vi "Automotive ECU - Park Brake.vi"() -> ()   [LabVIEW 2013]
doc: "Sample numeric display item."
uses:
  <vilib>/NI Veristand/Display Template Support/Display Template Support.llb/cluster_Screen Item Settings.ctl
  <vilib>/NI Veristand/Display Template Support/Display Template Support.llb/cluster_Graph Scale Settings.ctl
  <vilib>/NI Veristand/Display Template Support/Display Template Support.llb/cluster_Graph Plot Settings.ctl
  NationalInstruments.VeriStand.SystemStorage
  <vilib>/NI Veristand/Display Template Support/Display Template Support.llb/enum_Display Template Handler Minimal To Widget Msg.ctl
  <vilib>/NI Veristand/Display Template Support/Display Template Support.llb/enum_Display Template Handler Minimal To Workspace.ctl
  Support/Parking Brake Parameters.ctl
  <vilib>/NI Veristand/Execution/Workspace/NI_VS Workspace ExecutionAPI.lvlib
panel:
  in  "Parked":bool
  out "Label":string="Numeric"
  out "Status Indicator":string
  in  "NIVS.System Definition Root":refnum<k24>
  in  "NIVS.Gateway IP Address":string
  in  "Item.Data":T1
  # "Status:"
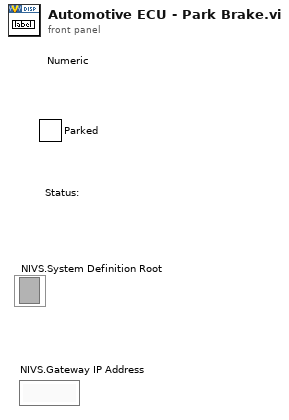
[diagram p1: front panel]
types:
  T1 = typedef "cluster_Screen Item Settings.ctl" = cluster{"Template VI":string, "Position X":i32, "Position Y":i32, "Custom":string, "Show Title Bar":bool, "ID":i32, "Always On Top":bool, "Allow Resize":bool, "Allow Minimize":bool, "Allow Close":bool, "Size to Screen":bool, "Screen.ID":i32, "State":enum16{"Normal", "New"}, "Title":string, "Window Bounds":cluster{"[0]":i16, "[1]":i16, "[2]":i16, "[3]":i16}, "Channel Ref":u64, "Unit":string, "Default Units?":bool, "Flash Limit?":bool, "Color 1":u32, "Color 2":u32, "Color 3":u32, "Color 4":u32, "Bck Color":u32, "Fore Color":u32, "Limit 1":dbl, "Limit 2":dbl, "Limit 3":dbl, "Limit 4":dbl, "Limit Mode 1":i32, "Limit Mode 2":i32, "Limit Mode 3":i32, "Limit Mode 4":i32, "Scale Precision":i32, "Scale Min":dbl, "Scale Max":dbl, "Format":i32, "Precision":i32, "Background Type":i32, "IDs":i32[], "Units":string[], "Labels":string[], "Scale Factor":dbl, "Scale Offset":dbl, "YScale Index":u32[], "XScale":T2, "YScales":T2[], "Plots":T3[], "Update Period":dbl, "History Length":dbl, "My.Ref":refnum<vi>, "Is Control?":bool, "Channel Paths":string[], "Custom Data":variant}
  T2 = typedef "cluster_Graph Scale Settings.ctl" = cluster{"Format":u8, "Precision":u8, "Fit":u8, "Label":string, "Use Default Label":bool, "Label Visible":bool, "Min":dbl, "Max":dbl}
  T3 = typedef "cluster_Graph Plot Settings.ctl" = cluster{"Bar Style":u8, "Fill To":i16, "Fill/PtColor":u32, "Line Style":u8, "Line Width":u8, "Color":u32, "Interp":u8, "Point Style":u8}
  T4 = typedef "enum_Display Template Handler Minimal To Workspace.ctl" = cluster{"Operation":enum16{"SetCustomData", "DeleteItem"}, "Data":variant}
  T5 = typedef "enum_Display Template Handler Minimal To Widget Msg.ctl" = enum16{"Stop", "LaunchConfigDialog"}
  T6 = typedef "Parking Brake Parameters.ctl" = cluster{"Ground on Engage":cluster{"Path Array":string[], "Node Path":string}, "Ground on Disengage":cluster{"Path Array":string[], "Node Path":string}, "Lower Pane Color":u32, "Upper Pane Color":u32, "Initialized?":bool, "Label":string}
  T7 = typedef "NI_VS Workspace ExecutionAPI.lvlib/WorkspaceAPI.ctl" = refnum<k24>
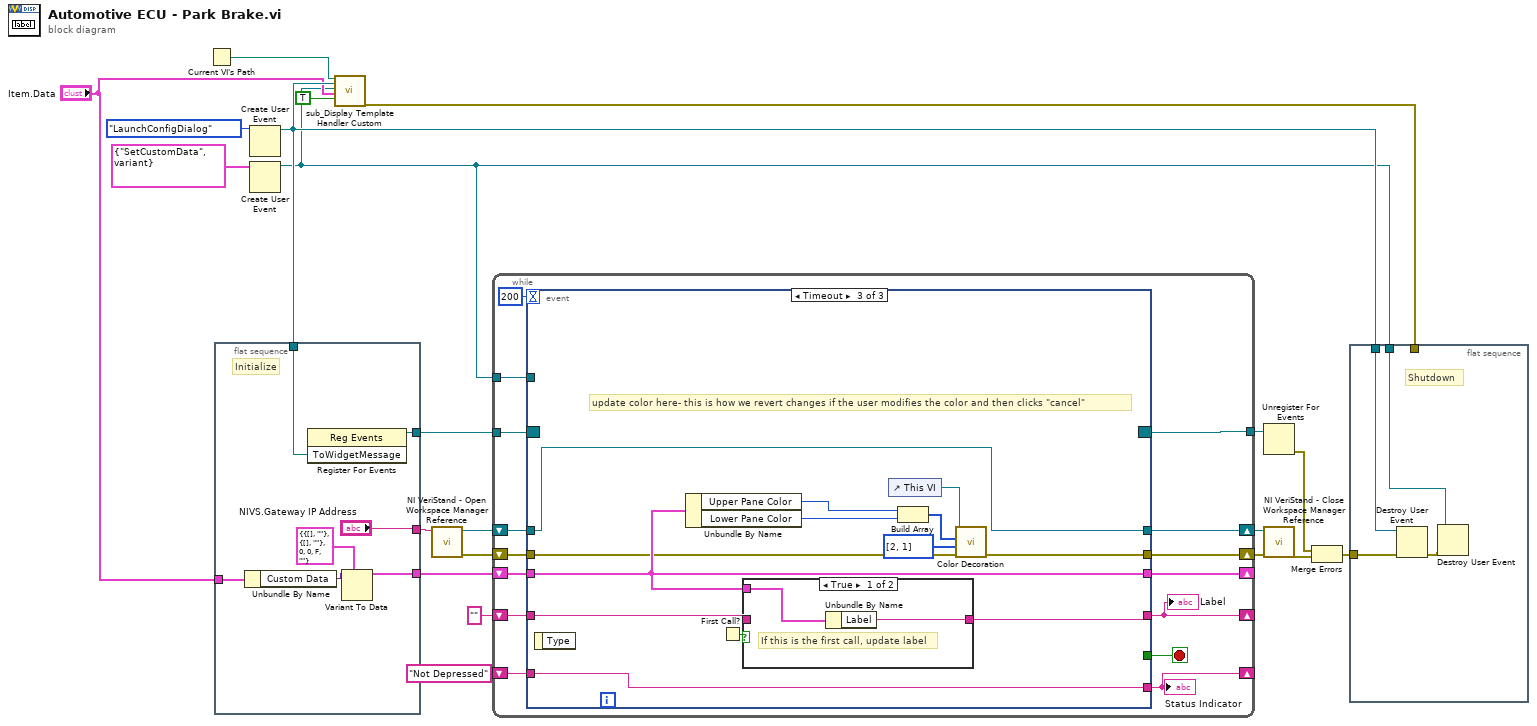
[diagram p0: block diagram]
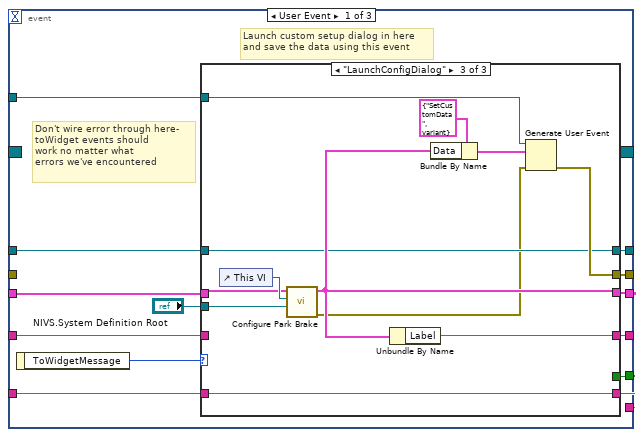
[diagram p2: hidden frame]
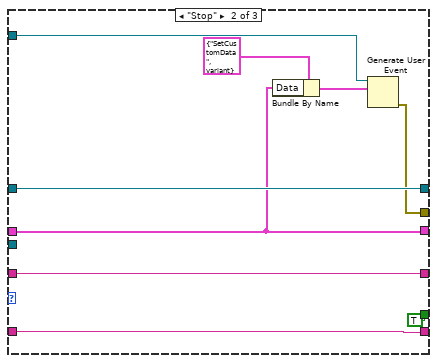
[diagram p4: hidden frame]
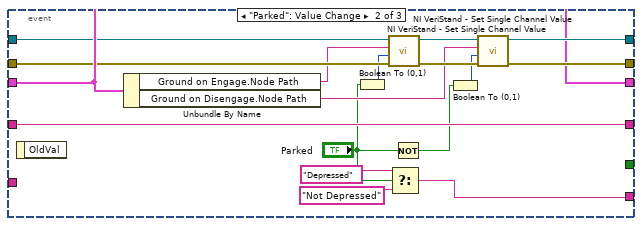
[diagram p5: hidden frame]
diagram:
  n1 = Current VI's Path() -> (path=w14:path)
  n2 = flat-sequence {
    tunnel: [w28] -> w19
    tunnel: w16 -> [w27]
    tunnel: "Item.Data" -> [w26]
    tunnel: [w23] -> w10
    tunnel: ["NIVS.Gateway IP Address"] -> w5
    frame #0 {
      # "Initialize"
      n3 = Unbundle By Name(w26) -> ("Custom Data"=w25:variant)
      n4 = register-events(w27) -> (reference out=w28:refnum<event-registration>)  [unwired: 2 in, 1 out]
      n5 = Variant To Data(type=T6 {"Ground on Engage"={"Path Array"=[], "Node Path"=""}, "Ground on Disengage"={"Path Array"=[], "Node Path"=""}, "Lower Pane Color"=0, "Upper Pane Color"=0, "Initialized?"=FALSE, "Label"=""} ("Park Brake Data in"), Variant=w25) -> (data=w23:T6)  [unwired: 1 in, 1 out]
    }
  }
  n6 = Create User Event(user event datatype=enum_Display_Template_Handler_Minimal_To_Widget_Msg."LaunchConfigDialog" ("ToWidgetMessage")) -> (user event=w16:refnum<user-event>)  [unwired: 1 in, 1 out]
  n7 = Create User Event(user event datatype=T4 {"Operation"=enum."SetCustomData", "Data"=variant} ("Data")) -> (user event=w12:refnum<user-event>)  [unwired: 1 in, 1 out]
  n8 = call <vilib>:"sub_Display Template Handler Custom.vi"("Parent.Path"=w14, "ToWidgetEvent"=w16, "ToWorkspace"=w12, "Item.Data"="Item.Data", "Resizable"=TRUE) -> ("error out"=w21:errorcluster)  [unwired: 14 in]
  n9 = call <vilib>:"NI VeriStand - Open Workspace Manager Reference.vi"("Gateway IP Address (\"\": localhost)"=w5) -> ("error out"=w8:errorcluster, "WorkspaceManager"=w9:T7)  [unwired: 9 in]
  n10 = while {
    tunnel: w19 -> [w43]
    tunnel: [w41] -> w18
    tunnel: w12 -> [w40]
    shift-right: [w32] -> _
    shift-left: w10 -> [w39]
    shift-right: [w36] -> w7
    shift-left: w9 -> [w38]
    shift-right: [w33] -> w6
    shift-left: w8 -> [w37]
    shift-right: [w34] -> _
    shift-left: "" ("Out") -> [w35]
    shift-right: [w30] -> _
    shift-left: "Not Depressed" -> [w29]
    stop <- w42 stop-if-true
    n11 = event shown="[2] Timeout" {
      selector: w43 -> [_ _ _]
      dyn-events: [_ _ _] -> w41
      timeout: 200 -> [_ _ _]
      tunnel: [w55 _ _] -> w42
      tunnel: w40 -> [w54 _ _]
      tunnel: w39 -> [w50 w95 w103]
      tunnel: w38 -> [w53 w92 w100]
      tunnel: w37 -> [_ w91 w102]
      tunnel: [w52 w97 w100] -> w36
      tunnel: [w48 w98 w101] -> w33
      tunnel: [w47 w96 w110] -> w34
      tunnel: w35 -> [w46 w96 w109]
      tunnel: [w49 w95 w103] -> w32
      tunnel: [w44 w82 w99] -> w30
      tunnel: w29 -> [w45 _ w99]
      event User Event {
        # "Don't wire error through here-\ntoWidget events should\nwork no matter what \nerrors we've encountered"
        # "Launch custom setup dialog in here\nand save the data using this event"
        n12 = event-data() -> ("ToWidgetMessage"=w56:T5)  [unwired: 1 out]
        n13 = case shown="\"LaunchConfigDialog\"" w56 {
          tunnel: [_ TRUE _] -> w55
          tunnel: w54 -> [_ w65 w78]
          tunnel: w53 -> [w60 w68 w72]
          tunnel: [w60 w68 w72] -> w52
          tunnel: "NIVS.System Definition Root" -> [_ _ w81]
          tunnel: w50 -> [w59 w64 w73]
          tunnel: [w59 w64 w77] -> w49
          tunnel: [_ w63 w76] -> w48
          tunnel: [w58 w62 w75] -> w47
          tunnel: w46 -> [w58 w62 _]
          tunnel: w45 -> [w57 w61 w70]
          tunnel: [w57 w61 w70] -> w44
          frame Default {
          }
          frame "Stop" {
            n14 = Bundle By Name(cluster=T4 {"Operation"=enum."SetCustomData", "Data"=variant} ("event data"), "Data"=w64) -> (w66:T4)
            n15 = Generate User Event(user event=w65, event data cluster=w66) -> (error out=w63:errorcluster)  [unwired: 2 in, 1 out]
          }
          frame "LaunchConfigDialog" {
            n16 = control-ref of="This VI"() -> (w74:refnum<vi>)
            n17 = call "Configure Park Brake.vi"("NIVS.System Definition Root"=w81, "VI Reference"=w74, "Park Brake Data in"=w73) -> ("error out"=w71:errorcluster, "Park Brake Data out"=w77:T6)  [unwired: 7 in]
            n18 = Unbundle By Name(w77) -> ("Label"=w75:string)
            n19 = Bundle By Name(cluster=T4 {"Operation"=enum."SetCustomData", "Data"=variant} ("event data"), "Data"=w77) -> (w80:T4)
            n20 = Generate User Event(user event=w78, event data cluster=w80, error in=w71) -> (error out=w76:errorcluster)  [unwired: 1 in, 1 out]
          }
        }
      }
      event "Parked": Value Change {
        n21 = event-data() -> ()  [unwired: 2 out]
        n22 = Unbundle By Name(w95) -> ("Ground on Engage.Node Path"=w90:string, "Ground on Disengage.Node Path"=w89:string)
        n23 = Boolean To (0,1)(Boolean="Parked") -> (0, 1=w88:i16)
        n24 = call <vilib>:"NI VeriStand - Set Single Channel Value.vi"("error in (no error)"=w91, "Value"=w88, "Channel"=w90, "WorkspaceManager in"=w92) -> ("error out"=w93:errorcluster, "WorkspaceManager out"=w94:T7)  [unwired: 6 in]
        n25 = Select(t="Depressed", s="Parked", f="Not Depressed") -> (s? t:f=w82:string)
        n26 = Not(x="Parked") -> (.not. x?=w87:bool)
        n27 = Boolean To (0,1)(Boolean=w87) -> (0, 1=w86:i16)
        n28 = call <vilib>:"NI VeriStand - Set Single Channel Value.vi"("error in (no error)"=w93, "Value"=w86, "Channel"=w89, "WorkspaceManager in"=w94) -> ("error out"=w98:errorcluster, "WorkspaceManager out"=w97:T7)  [unwired: 6 in]
      }
      event Timeout {
        # "update color here- this is how we revert changes if the user modifies the color and then clicks \"cancel\""
        n29 = event-data() -> ()  [unwired: 2 out]
        n30 = Unbundle By Name(w103) -> ("Upper Pane Color"=w107:u32, "Lower Pane Color"=w108:u32)
        n31 = First Call?() -> (First Call?: T/F=w111:bool)
        n32 = case shown="True" w111 {
          tunnel: w109 -> [_ w114]
          tunnel: [w112 w114] -> w110
          tunnel: w103 -> [w113 _]
          frame True {
            # "If this is the first call, update label"
            n33 = Unbundle By Name(w113) -> ("Label"=w112:string)
          }
          frame False {
            # "If this is the first call, update label"
          }
        }
        n34 = control-ref of="This VI"() -> (w106:refnum<vi>)
        n35 = Build Array(w107, w108) -> (w104:u32[])
        n36 = call "Color Decoration.vi"("VI reference"=w106, "Color Array"=w104, "Index Array"=u32[] [2, 1], "error in (no error)"=w102) -> ("error out"=w101:errorcluster)  [unwired: 6 in]
      }
    }
    "Label" <- w34
    "Status Indicator" <- w30
  }
  n37 = Unregister For Events(event registration refnum=w18) -> (error out=w17:errorcluster)  [unwired: 1 in]
  n38 = call <vilib>:"NI VeriStand - Close Workspace Manager Reference.vi"("error in (no error)"=w6, "WorkspaceManager"=w7) -> ("error out"=w1:errorcluster)  [unwired: 9 in]
  n39 = Merge Errors(w17, w1) -> (w2:errorcluster)
  n40 = flat-sequence {
    tunnel: w21 -> [_]
    tunnel: w2 -> [w117]
    tunnel: w16 -> [w118]
    tunnel: w12 -> [w115]
    frame #0 {
      # "Shutdown"
      n41 = Destroy User Event(user event=w118, error in=w117) -> (error out=w116:errorcluster)
      n42 = Destroy User Event(user event=w115, error in=w116) -> ()  [unwired: 1 out]
    }
  }
